vi "get runtime class name.vi"(8 "error in":errorcluster, 11 "Scan Engine configuration in":refnum<class "Scan Engine configuration.lvclass">) -> (0 "error out":errorcluster, 2 "class name":string, 3 "Scan Engine configuration out":refnum<class "Scan Engine configuration.lvclass">)   [LabVIEW 2013, in "Scan Engine configuration.lvclass"]
doc: "Provides an interface for determining the module runtime class associated with this module configuration. This class name can then be used to dynamically load or locate the runtime class for initialization purposes."
uses:
  Scan Engine configuration.lvclass
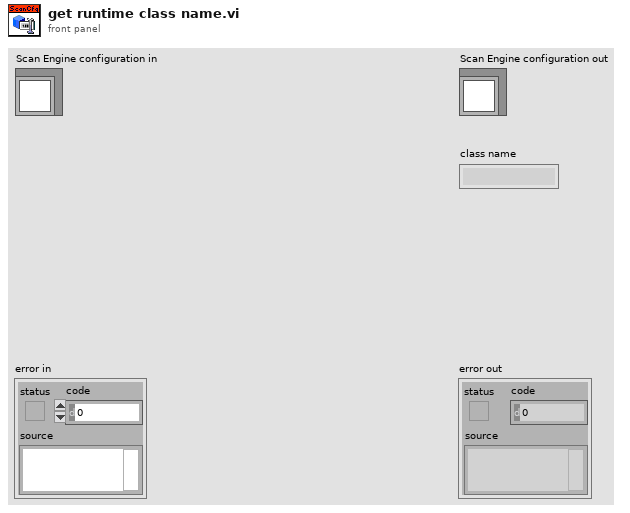
[diagram p1: front panel]
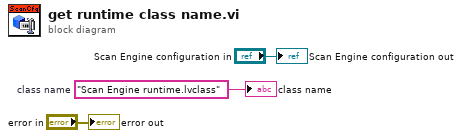
[diagram p0: block diagram]
diagram:
  w1 = "Scan Engine runtime.lvclass"  # class name
  "error out" <- "error in"
  "Scan Engine configuration out" <- "Scan Engine configuration in"
  "class name" <- w1
